vi "Measurement Logic.vi"(8 "error in":errorcluster, 9 "measurement configuration":T2={"Automation Test"=FALSE, "Power sequencing file path"="", "VST Resource Name"="5842_0", "RFSG port"="VNA-5633", "RFmx port"="", "RF Out Switch"="", "Common RFout"="", "Port1 Incident"="", "Port2 Incident"="", "RF In Switch"="", "Common RFin"="", "Port1 Reference"="", "Port1 Test"="", "Port2 Reference"="", "Port2 Test"="", "RFSG attenuation mode"=enum."Constant Attenuation", "RFSG external attenuation (dB)"=2.0, "Save Calibration File at"="", "Short S1P"="", "Open S1P"="", "Load S1P"="", "Through Adapter S2P"="", "Action"=enum."Measure", "Power Level (dBm)"=1.0, "External Gain (dB)"=2e-05, "Start Frequency (Hz)"=4000000000.0, "Stop Frequency (Hz)"=26000000000.0, "Step Size (Hz)"=0.0, "Type of Stimulus"=enum."Pulsed CW", "Pulse Width (s)"=1.0, "PRI (s)"=0.0, "IF Bandwidth (Hz)"=1.0, "Average Mode"=enum."Per Sweep", "Number of Averages"=0, "SnP File Path"="", "Calibration File Path"="", "Power sequencing file validity check"=TRUE} {"Step Size (Hz)" format="%#_6p"; "Stop Frequency (Hz)" format="%.3p"; "Start Frequency (Hz)" format="%.3p"; "Power Level (dBm)" format="%.2f"; "RFSG external attenuation (dB)" format="%.2f"}, 10 "measure call context in":refnum<class "Measure Call Context.lvclass">) -> (0 "error out":errorcluster, 1 "measurement results":T1, 2 "measure call context out":refnum<class "Measure Call Context.lvclass">)   [LabVIEW 2023, in "FPT_SParam_VST.lvclass"]
doc: "Contains the core logic for executing the measurement."
uses:
  FPT_SParam_VST.lvclass
  FPT_SParam_VST.lvclass/FPT_SParam_VST.ctl
  Measurement Configuration.ctl
  Measurement Results.ctl
  <vilib>/Analysis/NI_AALBase.lvlib
  <vilib>/Analysis/baseanly.llb/Mean (DBL).vi
  <vilib>/Plug-In SDKs/Measurements/Measure Call Context/Measure Call Context.lvclass
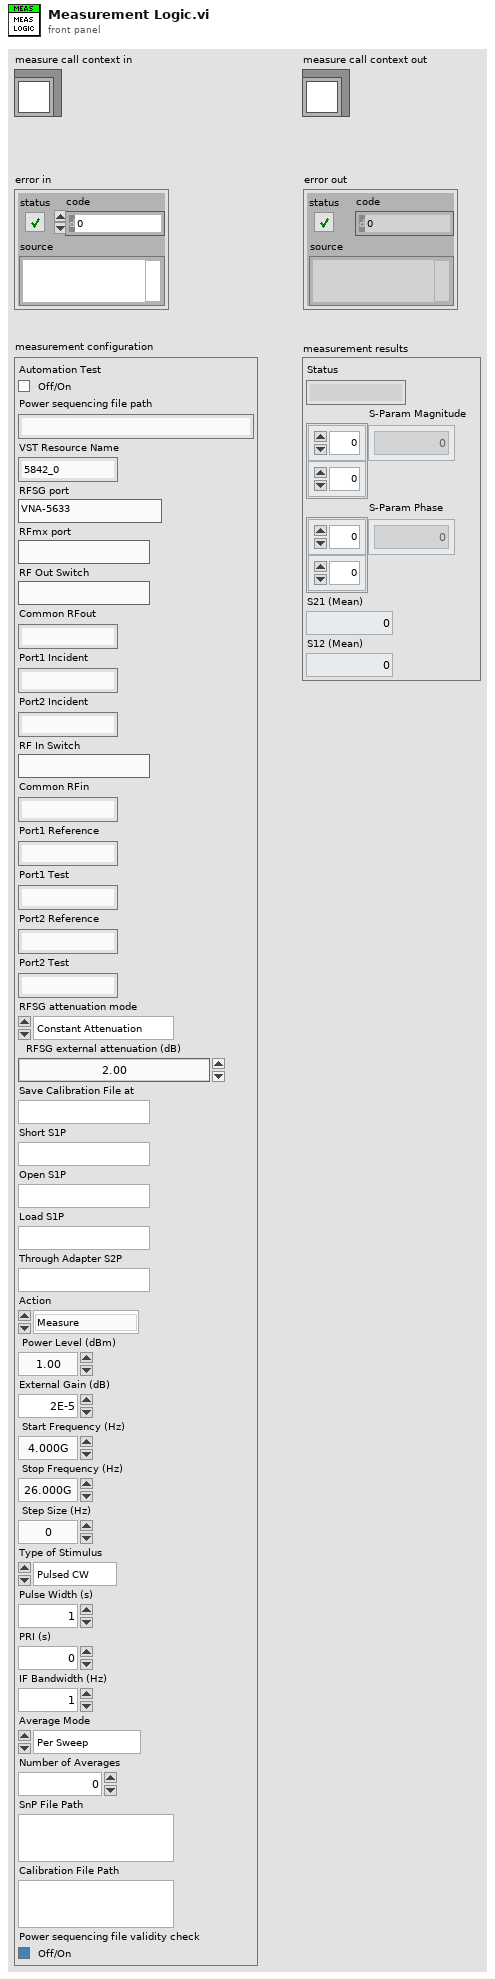
[diagram p1: front panel]
types:
  T1 = typedef "FPT_SParam_VST.lvclass/Measurement Results.ctl" = cluster{"Status":string, "S-Param Magnitude":dbl[][], "S-Param Phase":dbl[][], "S21 (Mean)":dbl, "S12 (Mean)":dbl}
  T2 = typedef "FPT_SParam_VST.lvclass/Measurement Configuration.ctl" = cluster{"Automation Test":bool, "Power sequencing file path":string, "VST Resource Name":string, "RFSG port":string, "RFmx port":string, "RF Out Switch":string, "Common RFout":string, "Port1 Incident":string, "Port2 Incident":string, "RF In Switch":string, "Common RFin":string, "Port1 Reference":string, "Port1 Test":string, "Port2 Reference":string, "Port2 Test":string, "RFSG attenuation mode":enum32{"<None>", "Constant Attenuation"}, "RFSG external attenuation (dB)":dbl, "Save Calibration File at":string, "Short S1P":string, "Open S1P":string, "Load S1P":string, "Through Adapter S2P":string, "Action":enum32{"Calibrate", "Measure"}, "Power Level (dBm)":dbl, "External Gain (dB)":dbl, "Start Frequency (Hz)":dbl, "Stop Frequency (Hz)":dbl, "Step Size (Hz)":dbl, "Type of Stimulus":enum32{"CW", "Pulsed CW"}, "Pulse Width (s)":dbl, "PRI (s)":dbl, "IF Bandwidth (Hz)":dbl, "Average Mode":enum32{"Per Sweep", "Per Point"}, "Number of Averages":i32, "SnP File Path":string, "Calibration File Path":string, "Power sequencing file validity check":bool}
  T3 = cluster{"measurement configuration":T2, "measurement results":T1, "CustomData":cluster{"Valid CSV":bool}}
  T4 = enum32{"Power On Dut", "Switching", "De-embedding + Measurement", "Power Off Dut"}[]
  T5 = typedef "Hardware Config - SParam_VST.ctl" = cluster{"VST Resource Name":refnum<k15>, "RFSG Port":string, "RFmx Port":string, "RF Out Switch":refnum<k15>, "RF Out Connection":cluster{"Common RFout":string, "Port1 Incident":string, "Port2 Incident":string}, "RF In Switch":refnum<k15>, "RF In Connection":cluster{"Common RFin":string, "Port1 Reference":string, "Port1 Test":string, "Port2 Reference":string, "Port2 Test":string}, "RFSG attenuation mode":enum32{"<None>", "Constant Attenuation"}, "RFSG Constant Attenuation (dB)":dbl, "Save Calibration File at":path, "Short S1P":path, "Open S1P":path, "Load S1P":path, "Through Adapter S2P":path}
  T6 = typedef "Test Config - SParam_VST.ctl" = cluster{"Action":enum32{"Calibrate", "Measure"}, "Power Level (dBm)":dbl, "External Gain (dB)":dbl, "Frequency Sweep":cluster{"Start Frequency (Hz)":dbl, "Stop Frequency (Hz)":dbl, "Step Size (Hz)":dbl}, "Type of Stimulus":enum16{"CW", "Pulsed CW"}, "Pulse Width (s)":dbl, "PRI (s)":dbl, "IF Bandwidth (Hz)":dbl, "Average Mode":enum16{"Per Sweep", "Per Point"}, "Number of Averages":i32, "SnP File Path":path, "Calibration File Path":path}
  T7 = typedef "Event Messenger-bool.lvlib/))Channel.ctl" = refnum<queue>
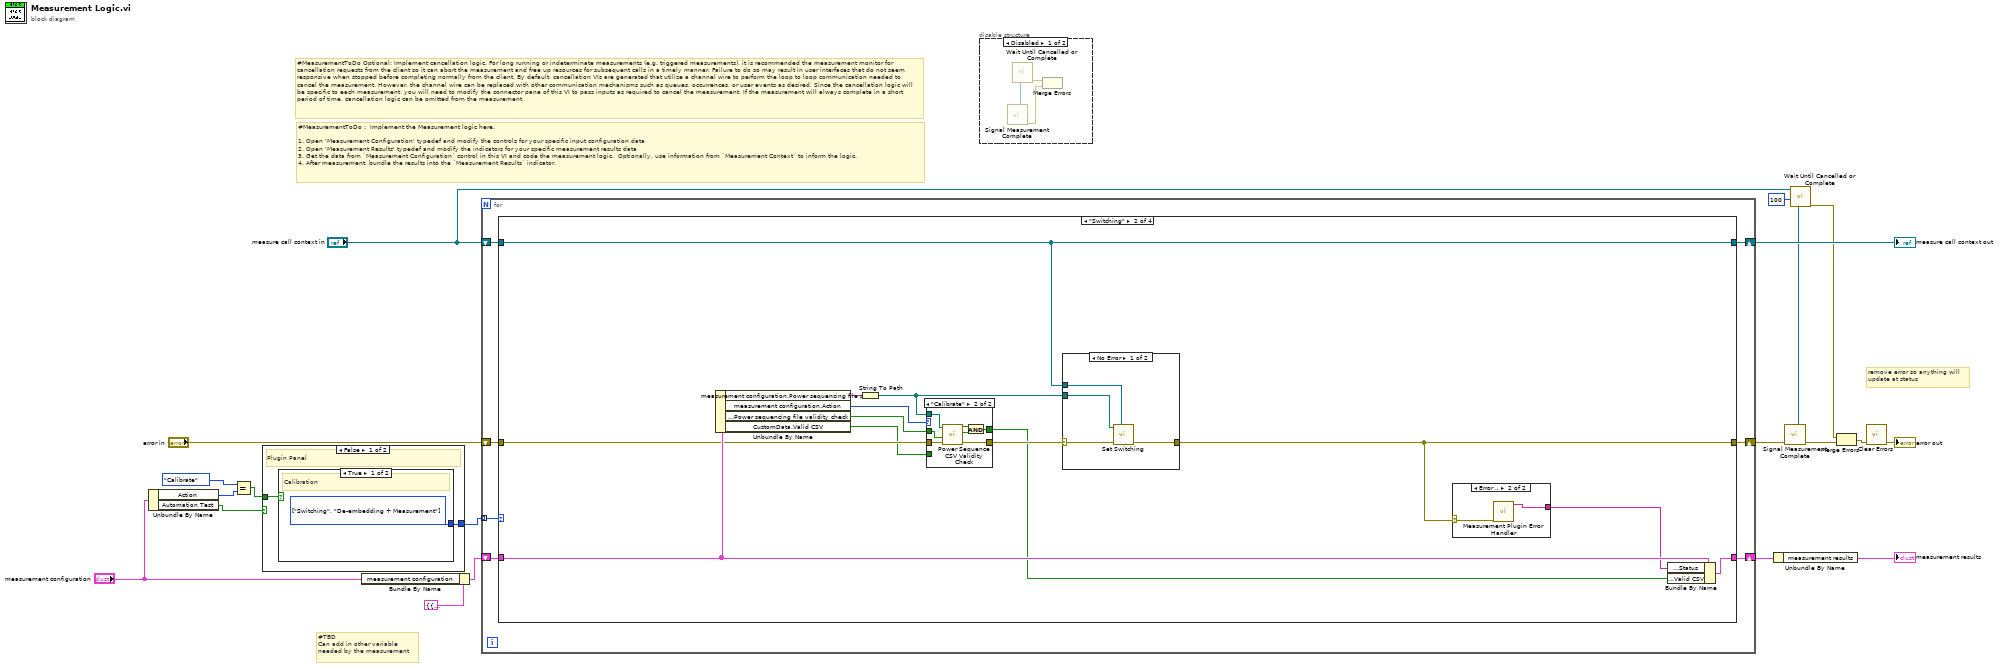
[diagram p0: block diagram]
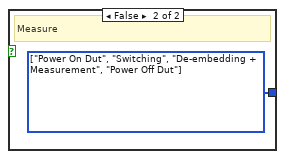
[diagram p2: hidden frame]
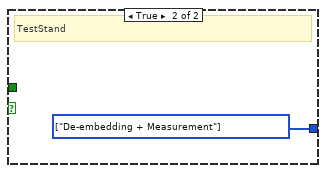
[diagram p3: hidden frame]
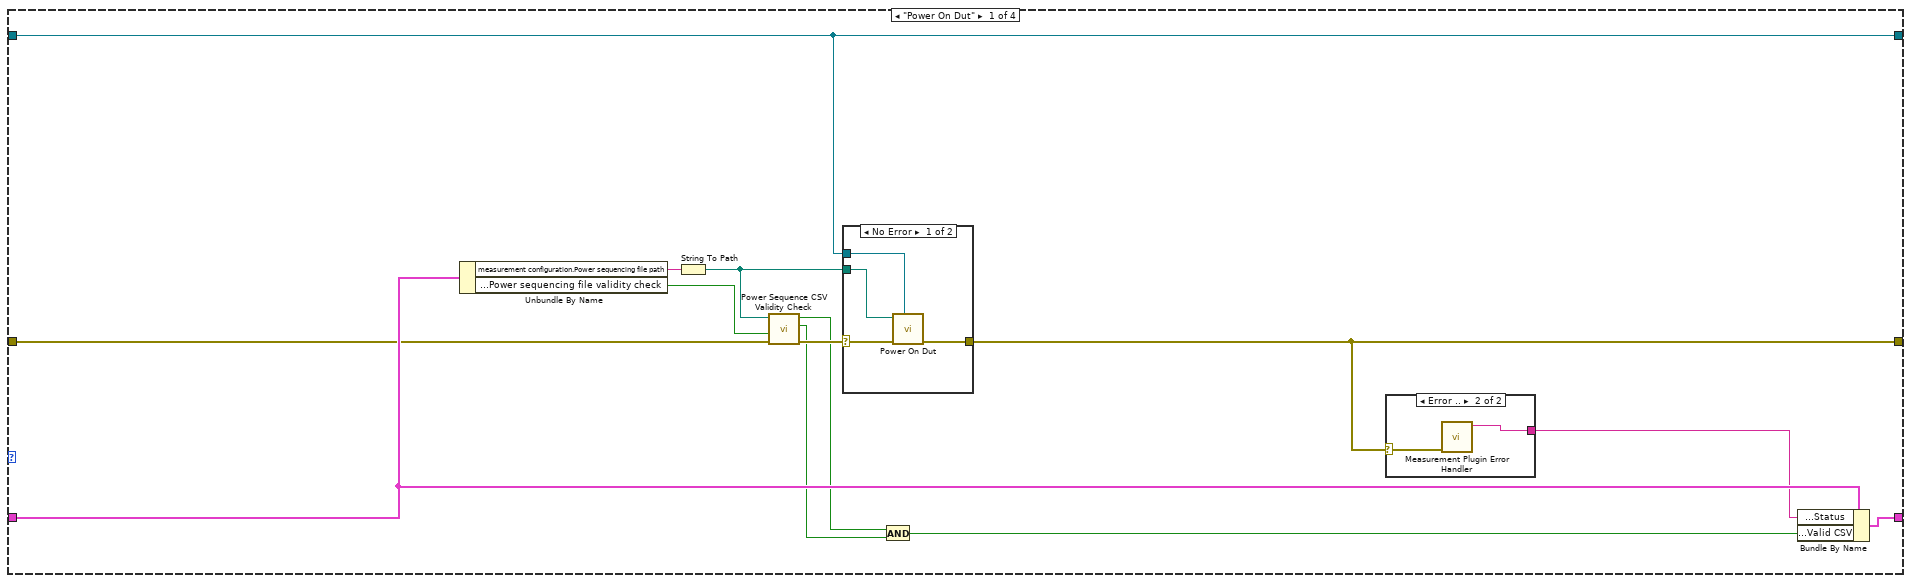
[diagram p4: hidden frame]
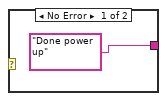
[diagram p6: hidden frame]
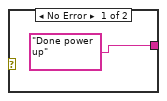
[diagram p9: hidden frame]
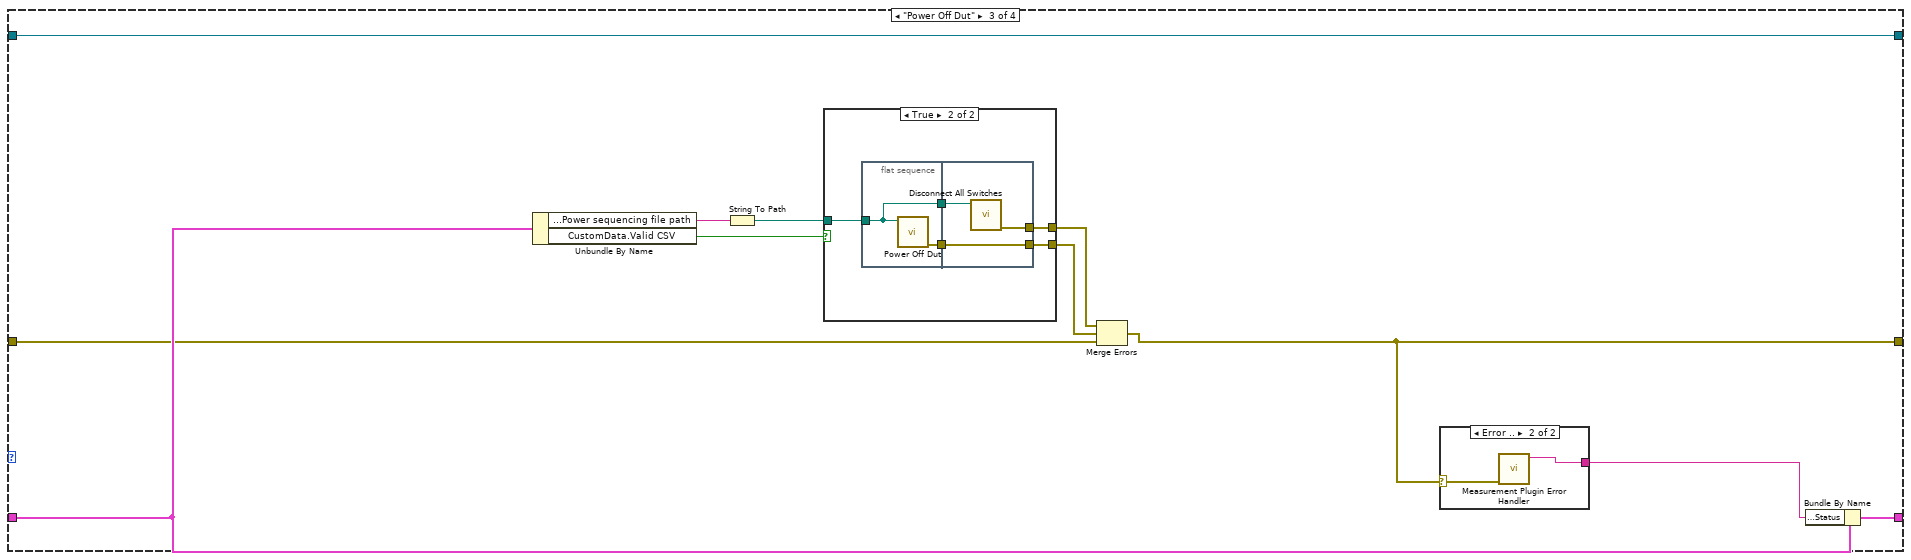
[diagram p10: hidden frame]
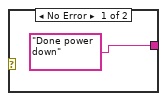
[diagram p12: hidden frame]
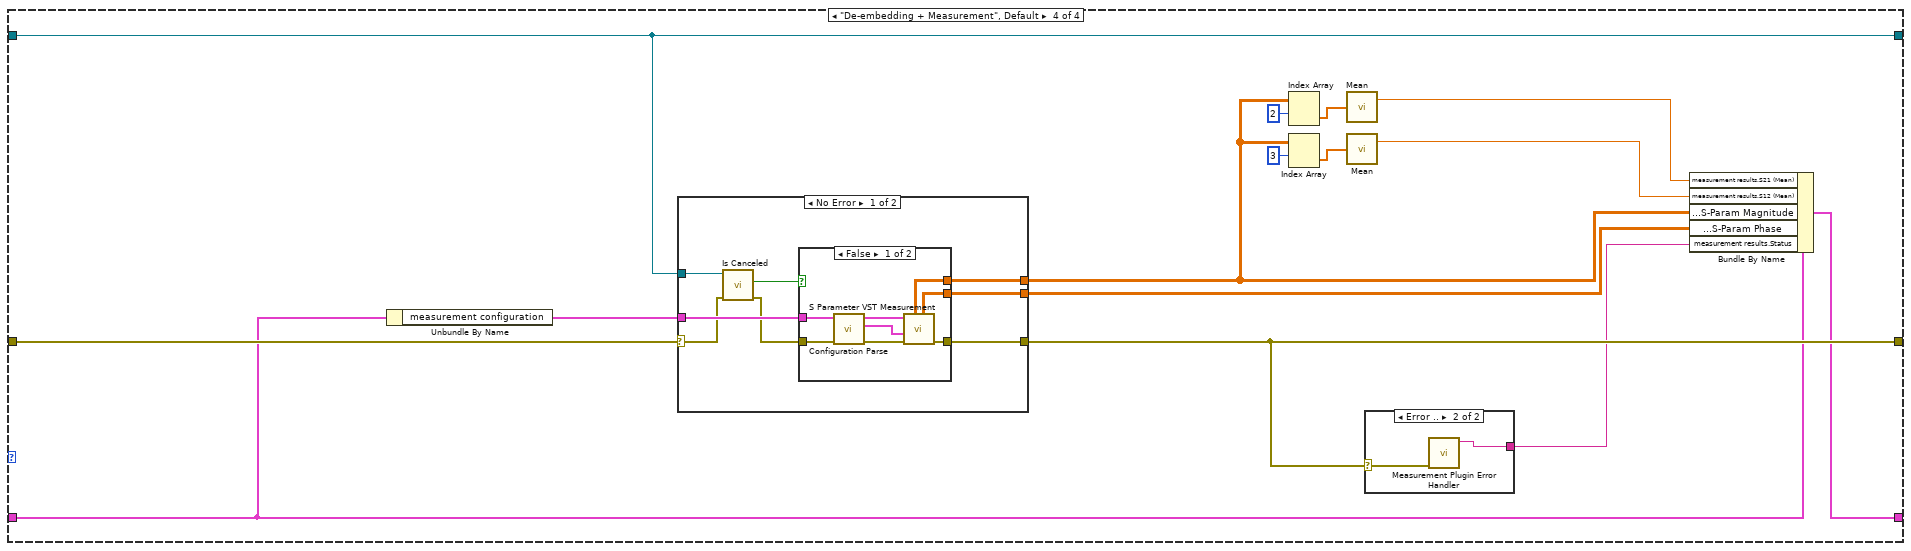
[diagram p13: hidden frame]
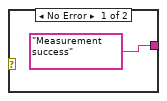
[diagram p14: hidden frame]
diagram:
  # "remove error so anything will\nupdate at status"
  # "#TBD\nCan add in other variable\nneeded by the measurement"
  # "#MeasurementToDo Optional: Implement cancellation logic. For long running or indeterminate measurements (e.g. triggered measurements), it is recommended the measurement monitor for cancellation requests from the client so it can abort the measurement and free up resources for subsequent calls in a timely manner. Failure to do so may result in user interfaces that do not seem responsive when stopped before completing normally from the client. By default, cancellation VIs are generated that utilize a channel wire to perform the loop to loop communication needed to cancel the measurement. However, the channel wire can be replaced with other communication mechanisms such as queues, occurrences, or user events as desired. Since the cancellation logic will be specific to each measurement, you will need to modify the connector pane of this VI to pass inputs as required to cancel the measurement. If the measurement will always complete in a short period of time, cancellation logic can be omitted from the measurement."
  # "#MeasurementToDo :  Implement the Measurement logic here.\n\n1. Open 'Measurement Configuration' typedef and modify the controls for your specific input configuration data\n2. Open 'Measurement Results' typedef and modify the indicators for your specific measurement results data\n3. Get the data from `Measurement Configuration` control in this VI and code the measurement logic.  Optionally, use information from `Measurement Context` to inform the logic.\n4. After measurement, bundle the results into the `Measurement Results` indicator."
  n1 = Unbundle By Name("measurement configuration") -> ("Action"=w10:enum32{"Calibrate", "Measure"}, "Automation Test"=w11:bool)
  n2 = Equal?(x=enum32{"Calibrate", "Measure"}."Calibrate", y=w10) -> (x = y?=w9:bool)
  n3 = case shown="False" w11 {
    tunnel: [w22 w25] -> w12
    tunnel: w9 -> [w21 _]
    frame False {
      # "Plugin Panel"
      n4 = case shown="True" w21 {
        tunnel: [w23 w24] -> w22
        frame True {
          w23 = T4 [enum."Switching", enum."De-embedding + Measurement"] items=["Power On Dut", "Switching", "De-embedding + Measurement", "Power Off Dut"]
          # "Calibration"
        }
        frame False {
          w24 = T4 [enum."Power On Dut", enum."Switching", enum."De-embedding + Measurement", enum."Power Off Dut"] items=["Power On Dut", "Switching", "De-embedding + Measurement", "Power Off Dut"]
          # "Measure"
        }
      }
    }
    frame True {
      w25 = T4 [enum."De-embedding + Measurement"] items=["Power On Dut", "Switching", "De-embedding + Measurement", "Power Off Dut"]
      # "TestStand"
    }
  }
  n5 = Bundle By Name(cluster=T3 {"measurement configuration"={"Automation Test"=FALSE, "Power sequencing file path"="", "VST Resource Name"="5842_0", "RFSG port"="VNA-5633", "RFmx port"="", "RF Out Switch"="", "Common RFout"="", "Port1 Incident"="", "Port2 Incident"="", "RF In Switch"="", "Common RFin"="", "Port1 Reference"="", "Port1 Test"="", "Port2 Reference"="", "Port2 Test"="", "RFSG attenuation mode"=enum."Constant Attenuation", "RFSG external attenuation (dB)"=2.0, "Save Calibration File at"="", "Short S1P"="", "Open S1P"="", "Load S1P"="", "Through Adapter S2P"="", "Action"=enum."Measure", "Power Level (dBm)"=1.0, "External Gain (dB)"=2e-05, "Start Frequency (Hz)"=4000000000.0, "Stop Frequency (Hz)"=26000000000.0, "Step Size (Hz)"=0.0, "Type of Stimulus"=enum."Pulsed CW", "Pulse Width (s)"=1.0, "PRI (s)"=0.0, "IF Bandwidth (Hz)"=1.0, "Average Mode"=enum."Per Sweep", "Number of Averages"=0, "SnP File Path"="", "Calibration File Path"="", "Power sequencing file validity check"=TRUE}, "measurement results"={"Status"="", "S-Param Magnitude"=[], "S-Param Phase"=[], "S21 (Mean)"=0.0, "S12 (Mean)"=0.0}, "CustomData"={"Valid CSV"=FALSE}}, "measurement configuration"="measurement configuration") -> (w18:T3)
  n6 = for {
    tunnel: w12 -> [w31] mode=indexing
    shift-right: [w26] -> w1
    shift-left: "error in" -> [w32]
    shift-right: [w27] -> w16
    shift-left: w18 -> [w30]
    shift-right: [w28] -> w17
    shift-left: "measure call context in" -> [w29]
    n7 = case shown="\"Switching\"" w31 {
      tunnel: w32 -> [w39 w60 w88 w118]
      tunnel: w30 -> [w45 w66 w90 w117]
      tunnel: w29 -> [w40 w61 w93 w109]
      tunnel: [w41 w62 w89 w122] -> w26
      tunnel: [w40 w61 w93 w109] -> w28
      tunnel: [w43 w64 w91 w120] -> w27
      frame "Power On Dut" {
        n8 = Unbundle By Name(w45) -> ("measurement configuration.Power sequencing file path"=w42:string, "measurement configuration.Power sequencing file validity check"=w36:bool)
        n9 = String To Path(string=w42) -> (path=w38:path)
        n10 = call "Power Sequence CSV Validity Check.vi"("error in"=w39, "Enable Validity Check?"=w36, "File Path"=w38) -> ("error out"=w37:errorcluster, "Valid Execution Order"=w34:bool, "All Instruments Available"=w35:bool)  [unwired: 5 in, 1 out]
        n11 = case shown="No Error" w37 {
          selector: w37 -> [w46 w50]
          tunnel: [w49 w50] -> w41
          tunnel: w40 -> [w48 _]
          tunnel: w38 -> [w47 _]
          frame No Error {
            n12 = call "Power On Dut.vi"("measure call context in"=w48, "error in"=w46, "Power sequencing file path"=w47) -> ("error out"=w49:errorcluster)  [unwired: 7 in, 1 out]
          }
          frame Error {
          }
        }
        n13 = And(x=w35, y=w34) -> (x .and. y?=w33:bool)
        n14 = case shown="Error .." w41 {
          selector: w41 -> [_ w53]
          tunnel: ["Done power up" w52] -> w44
          frame No Error {
          }
          frame Error {
            n15 = call "Measurement Plugin Error Handler.vi"("error in"=w53) -> ("Status Message (Error)"=w52:string)  [unwired: 9 in, 1 out]
          }
        }
        n16 = Bundle By Name(cluster=w45, "measurement results.Status"=w44, "CustomData.Valid CSV"=w33) -> (w43:T3)
      }
      frame "Switching" {
        n17 = Unbundle By Name(w66) -> ("measurement configuration.Power sequencing file path"=w63:string, "measurement configuration.Action"=w58:enum32{"Calibrate", "Measure"}, "measurement configuration.Power sequencing file validity check"=w56:bool, "CustomData.Valid CSV"=w55:bool)
        n18 = String To Path(string=w63) -> (path=w57:path)
        n19 = case shown="\"Calibrate\"" w58 {
          tunnel: w60 -> [w68 w75]
          tunnel: [w68 w74] -> w59
          tunnel: w57 -> [_ w73]
          tunnel: w56 -> [_ w72]
          tunnel: w55 -> [w67 _]
          tunnel: [w67 w69] -> w54
          frame Default {
          }
          frame "Calibrate" {
            n20 = call "Power Sequence CSV Validity Check.vi"("error in"=w75, "Enable Validity Check?"=w72, "File Path"=w73) -> ("error out"=w74:errorcluster, "Valid Execution Order"=w70:bool, "All Instruments Available"=w71:bool)  [unwired: 5 in, 1 out]
            n21 = And(x=w71, y=w70) -> (x .and. y?=w69:bool)
          }
        }
        n22 = case shown="No Error" w59 {
          selector: w59 -> [w76 w80]
          tunnel: [w79 w80] -> w62
          tunnel: w57 -> [w78 _]
          tunnel: w61 -> [w77 _]
          frame No Error {
            n23 = call "Set Switching.vi"("measure call context in"=w77, "error in"=w76, "File Path"=w78) -> ("error out"=w79:errorcluster)  [unwired: 7 in, 1 out]
          }
          frame Error {
          }
        }
        n24 = case shown="Error .." w62 {
          selector: w62 -> [_ w83]
          tunnel: ["Done power up" w82] -> w65
          frame No Error {
          }
          frame Error {
            n25 = call "Measurement Plugin Error Handler.vi"("error in"=w83) -> ("Status Message (Error)"=w82:string)  [unwired: 9 in, 1 out]
          }
        }
        n26 = Bundle By Name(cluster=w66, "measurement results.Status"=w65, "CustomData.Valid CSV"=w54) -> (w64:T3)
      }
      frame "Power Off Dut" {
        n27 = Unbundle By Name(w90) -> ("measurement configuration.Power sequencing file path"=w94:string, "CustomData.Valid CSV"=w84:bool)
        n28 = String To Path(string=w94) -> (path=w85:path)
        n29 = case shown="True" w84 {
          tunnel: [_ w97] -> w87
          tunnel: [_ w96] -> w86
          tunnel: w85 -> [_ w95]
          frame False {
          }
          frame True {
            n30 = flat-sequence {
              tunnel: w95 -> [w100]
              tunnel: [w101] -> w99
              tunnel: [w100] -> w98
              tunnel: [w104] -> w97
              tunnel: w99 -> [w104]
              tunnel: [w103] -> w96
              tunnel: w98 -> [w102]
              frame #0 {
                n31 = call "Power Off Dut.vi"("Power Sequencing File Path"=w100) -> ("error out"=w101:errorcluster)  [unwired: 10 in]
              }
              frame #1 {
                n32 = call "Disconnect All Switches.vi"("File Path"=w102) -> ("error out"=w103:errorcluster)  [unwired: 10 in]
              }
            }
          }
        }
        n33 = Merge Errors(w86, w87, w88) -> (w89:errorcluster)
        n34 = case shown="Error .." w89 {
          selector: w89 -> [_ w107]
          tunnel: ["Done power down" w106] -> w92
          frame No Error {
          }
          frame Error {
            n35 = call "Measurement Plugin Error Handler.vi"("error in"=w107) -> ("Status Message (Error)"=w106:string)  [unwired: 9 in, 1 out]
          }
        }
        n36 = Bundle By Name(cluster=w90, "measurement results.Status"=w92) -> (w91:T3)
      }
      frame "De-embedding + Measurement", Default {
        n37 = Unbundle By Name(w117) -> ("measurement configuration"=w108:T2)
        n38 = case shown="No Error" w118 {
          selector: w118 -> [w129 w143]
          tunnel: [w133 w143] -> w122
          tunnel: [w131 _] -> w112
          tunnel: [w130 _] -> w119
          tunnel: w108 -> [w132 _]
          tunnel: w109 -> [w126 _]
          frame No Error {
            n39 = call <vilib>:"Is Canceled.vi"("error in"=w129, "measure call context in"=w126) -> ("error out"=w128:errorcluster, "is canceled?"=w127:bool)  [unwired: 7 in, 1 out]
            n40 = case shown="False" w127 {
              tunnel: [w141 w142] -> w133
              tunnel: w132 -> [w137 _]
              tunnel: w128 -> [w136 w142]
              tunnel: [w135 _] -> w131
              tunnel: [w134 _] -> w130
              frame False {
                n41 = call "Configuration Parse.vi"("error in"=w136, "Measurement Configuration"=w137) -> ("error out"=w139:errorcluster, "RFmxVNA Settings"=w140:T5, "Test Configuration"=w138:T6)  [unwired: 7 in]
                n42 = call "S Parameter VST Measurement.vi"("error in"=w139, "SPML Settings"=w140, "Test Configuration"=w138) -> ("error out"=w141:errorcluster, "S-Param Phase"=w134:dbl[][], "S-Param Magnitude"=w135:dbl[][])  [unwired: 6 in]
              }
              frame True {
              }
            }
          }
          frame Error {
          }
        }
        n43 = Index Array(array=w112, index (row)=2) -> (element=w116:dbl[])  [unwired: 1 in]
        n44 = Index Array(array=w112, index (row)=3) -> (element=w115:dbl[])  [unwired: 1 in]
        n45 = call-poly <vilib>:"Mean.vi"("X"=w116) -> ("mean"=w111:dbl)  [unwired: 1 out]
        n46 = call-poly <vilib>:"Mean.vi"("X"=w115) -> ("mean"=w110:dbl)  [unwired: 1 out]
        n47 = case shown="Error .." w122 {
          selector: w122 -> [_ w125]
          tunnel: ["Measurement success" w124] -> w121
          frame No Error {
          }
          frame Error {
            n48 = call "Measurement Plugin Error Handler.vi"("error in"=w125) -> ("Status Message (Error)"=w124:string)  [unwired: 9 in, 1 out]
          }
        }
        n49 = Bundle By Name(cluster=w117, "measurement results.S21 (Mean)"=w111, "measurement results.S12 (Mean)"=w110, "measurement results.S-Param Magnitude"=w112, "measurement results.S-Param Phase"=w119, "measurement results.Status"=w121) -> (w120:T3)
      }
    }
  }
  "measure call context out" <- w17
  n50 = disable-structure shown="Disabled" {
    frame Disabled {
      n51 = call "Signal Measurement Complete.vi"() -> ("error out"=w145:errorcluster, "done channel"=w146:T7)  [unwired: 10 in]
      n52 = call "Wait Until Cancelled or Complete.vi"("done channel"=w146) -> ("error out"=w144:errorcluster)  [unwired: 9 in, 1 out]
      n53 = Merge Errors(w144, w145) -> ()  [unwired: 1 out]
    }
    frame Enabled {
    }
  }
  n54 = Unbundle By Name(w16) -> ("measurement results"=→"measurement results":T1)
  n55 = call "Signal Measurement Complete.vi"("error in (no error)"=w1) -> ("error out"=w2:errorcluster, "done channel"=w3:T7)  [unwired: 9 in]
  n56 = call "Wait Until Cancelled or Complete.vi"("done channel"=w3, "ms polling interval"=100, "measure call context in"="measure call context in") -> ("error out"=w4:errorcluster)  [unwired: 7 in, 1 out]
  n57 = Merge Errors(w4, w2) -> (w5:errorcluster)
  n58 = call <vilib>:"Clear Errors.vi"("error in (no error)"=w5) -> ("error out"=→"error out":errorcluster)  [unwired: 5 in, 1 out]
